vi "Vertical Rod Sensor-State converter.vi"(0 "UP Sensor":bool, 2 "DOWN Sensor":bool) -> (7 "Status":T1)   [LabVIEW 2016]
doc: "Takes UP/DOWN sensor data and converts to state of vertical (sample) rod:\n\nUP = TRUE; DOWN = FALSE --> State = \"rod up\"\nUP = TRUE; DOWN = TRUE --> State = \"status unclear\"\nUP = FALSE; DOWN = TRUE --> State = \"rod down\"\nUP = FALSE; DOWN = FALSE --> State = \"status unclear\""
uses:
  controls/Vertical Rod states.ctl
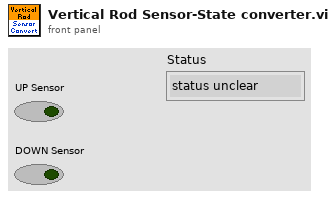
[diagram p1: front panel]
types:
  T1 = typedef "Vertical Rod states.ctl" = enum16{"status unclear", "rod down", "rod up"}
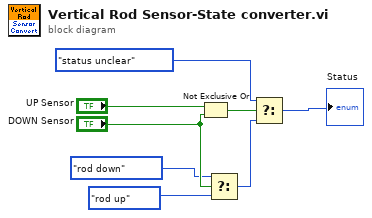
[diagram p0: block diagram]
diagram:
  n1 = Not Exclusive Or(1:"DOWN Sensor", 2:"UP Sensor") -> (0:w5:bool)
  n2 = Select(t=Vertical_Rod_states."rod down" ("Enum"), s="DOWN Sensor", f=Vertical_Rod_states."rod up" ("Enum")) -> (s? t:f=w7:T1)
  n3 = Select(t=Vertical_Rod_states."status unclear" ("Enum"), s=w5, f=w7) -> (s? t:f=→"Status":T1)
